vi "IR_Ttest.vi"(1 "inData":string[](array[string])) -> (15 "OutData":string[](array[string]), 16 "结果数组":bool[](array[boolean]), 17 "读取缓冲区":string)   [LabVIEW 2018]
uses:
  Subvi/Global.vi
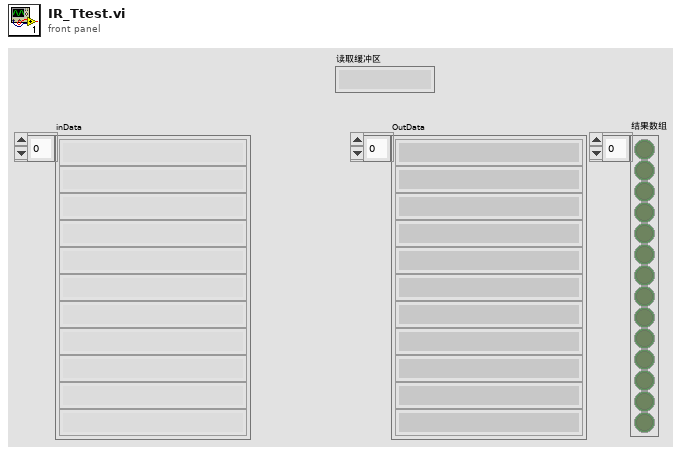
[diagram p1: front panel]
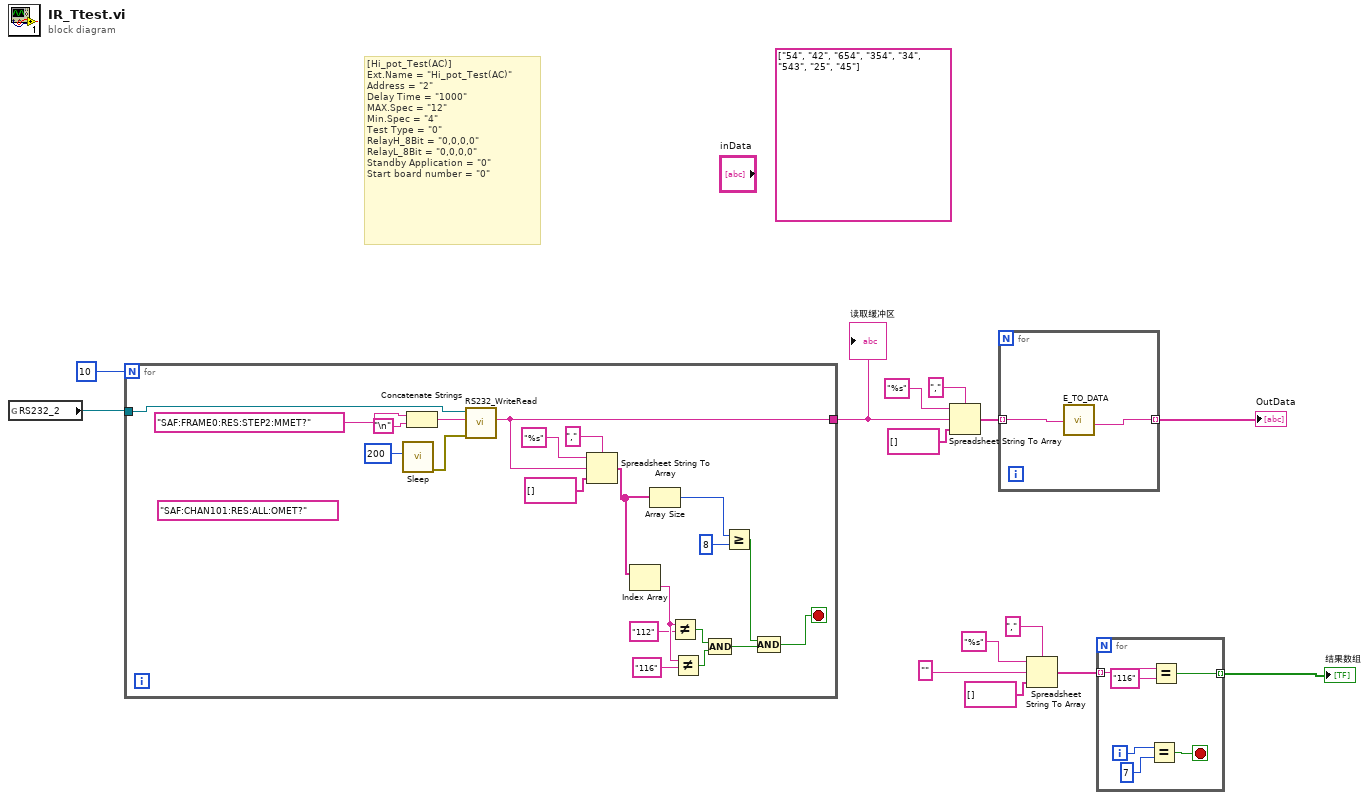
[diagram p0: block diagram]
diagram:
  (unwired) string[] ["54", "42", "654", "354", "34", "543", "25", "45"]
  # "[Hi_pot_Test(AC)]\nExt.Name = \"Hi_pot_Test(AC)\"\nAddress = \"2\"\nDelay Time = \"1000\"\nMAX.Spec = \"12\"\nMin.Spec = \"4\"\nTest Type = \"0\"\nRelayH_8Bit = \"0,0,0,0\"\nRelayL_8Bit = \"0,0,0,0\"\nStandby Application = \"0\"\nStart board number = \"0\""
  n1 = global read "Global.vi" "RS232_2"() -> (w14:refnum<visa-resource-name>)
  n2 = for {
    N: 10 -> [_]
    tunnel: [w26] -> w13
    tunnel: w14 -> [w35]
    stop <- w15 stop-if-true
    (unwired) "SAF:CHAN101:RES:ALL:OMET?" ("写入缓冲区")
    n3 = call "Sleep.vi"("等待时间（毫秒）"=u32 200) -> ("error out"=w31:errorcluster)  [unwired: 10 in]
    n4 = Concatenate Strings("SAF:FRAME0:RES:STEP2:MMET?" ("写入缓冲区"), "\n") -> (w34:string)
    n5 = call "RS232_WriteRead.vi"("错误输入（无错误）"=w31, "写入缓冲区"=w34, "VISA资源名称"=w35) -> ("读取缓冲区"=w26:string)  [unwired: 6 in, 2 out]
    n6 = Spreadsheet String To Array(delimiter (Tab)="," ("分隔符(Tab)"), format string="%s" ("电子表格字符串"), spreadsheet string=w26, array type (2D Dbl)=string[] []) -> (array=w17:string[])
    n7 = Index Array(array=w17) -> (element=w23:string)  [unwired: 1 in]
    n8 = Array Size(array=w17) -> (size(s)=w25:i32)
    n9 = Not Equal?(x=w23, y="112") -> (x != y?=w22:bool)
    n10 = Not Equal?(x=w23, y="116") -> (x != y?=w21:bool)
    n11 = Compound Arithmetic op=AND ("复合运算")(w22, w21) -> (w20:bool)
    n12 = Greater Or Equal?(x=w25, y=8) -> (x >= y?=w16:bool)
    n13 = Compound Arithmetic op=AND ("复合运算")(w16, w20) -> (w15:bool)
  }
  "读取缓冲区" <- w13
  n14 = Spreadsheet String To Array(delimiter (Tab)="," ("分隔符(Tab)"), format string="%s" ("电子表格字符串"), spreadsheet string=w13, array type (2D Dbl)=string[] []) -> (array=w2:string[])
  n15 = for {
    tunnel: w2 -> [w37] mode=indexing
    tunnel: [w36] -> w1 mode=indexing
    n16 = call "E_TO_DATA.vi"("INPUT"=w37) -> ("子字符串"=w36:string)  [unwired: 9 in, 1 out]
  }
  "OutData" <- w1
  n17 = Spreadsheet String To Array(delimiter (Tab)="," ("分隔符(Tab)"), format string="%s" ("电子表格字符串"), spreadsheet string="" ("电子表格字符串"), array type (2D Dbl)=string[] []) -> (array=w9:string[])
  n18 = for {
    tunnel: w9 -> [w40] mode=indexing
    tunnel: [w38] -> w5 mode=indexing
    i -> [w42]
    stop <- w41 stop-if-true
    n19 = Equal?(x=w42, y=7) -> (x = y?=w41:bool)
    n20 = Equal?(x=w40, y="116") -> (x = y?=w38:bool)
  }
  "结果数组" <- w5
